vi "SLSC Create VS Channels.vi"(11 "Array in":T1(array[cluster])) -> (3 "Array out":T2[](array[typedef]))   [LabVIEW 2019, in "SLSC-12201 DIO System Explorer.lvlib"]
uses:
  SLSC-12201 DIO System Explorer.lvlib
  Shared/SLSC Channel Information.ctl
  <vilib>/NI VeriStand/Custom Device API/Custom Device Channel.ctl
  <vilib>/NI VeriStand/Custom Device API/Custom Device Channel Type.ctl
  <vilib>/NI VeriStand/Custom Device API/Custom Device API.lvlib
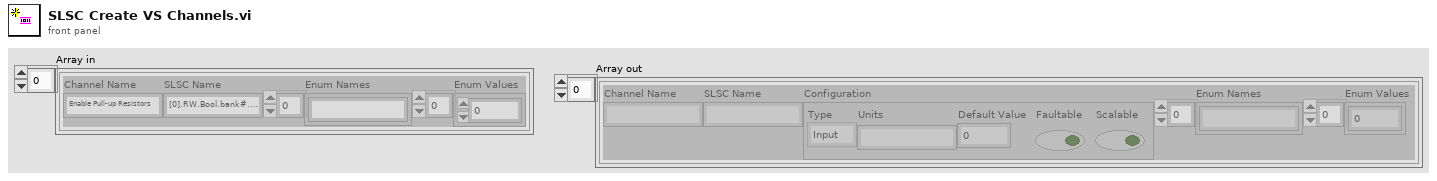
[diagram p1: front panel]
types:
  T1 = cluster{"Channel Name":string, "SLSC Name":string, "Enum Names":string[], "Enum Values":i32[]}[]
  T2 = typedef "SLSC-12201 DIO System Explorer.lvlib/SLSC Channel Information.ctl" = cluster{"Channel Name":string, "SLSC Name":string, "Configuration":T3, "Enum Names":string[], "Enum Values":i32[]}
  T3 = typedef "Custom Device API.lvlib/Custom Device Channel.ctl" = cluster{"Type":T4, "Units":string, "Default Value":dbl, "Faultable":bool, "Scalable":bool}
  T4 = typedef "Custom Device API.lvlib/Custom Device Channel Type.ctl" = enum16{"Input", "Output"}
  T5 = cluster{"Channel Name":string, "Channel ":string, "output cluster":T3, "Enum Names":string[], "Enum Values":i32[]}
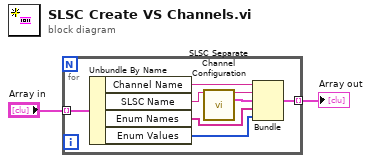
[diagram p0: block diagram]
diagram:
  n1 = for {
    tunnel: "Array in" -> [w10] mode=indexing
    tunnel: [w5] -> w1 mode=indexing
    n2 = Unbundle By Name(w10) -> ("Channel Name"=w9:string, "SLSC Name"=w8:string, "Enum Names"=w4:string[], "Enum Values"=w3:i32[])
    n3 = call "SLSC Separate Channel Configuration.vi"("Encoded String"=w8) -> ("Channel"=w7:string, "output cluster"=w6:T3)  [unwired: 9 in, 4 out]
    n4 = Bundle("Channel Name"=w9, "Channel"=w7, "output cluster"=w6, "Enum Names"=w4, "Enum Values"=w3) -> (w5:T5)  [unwired: 1 in]
  }
  "Array out" <- w1
